vi "ERROR HANDLER.vi"(2 "error in":T1, 3 "GPIB address":string="8") -> (0 "error out":T1, 1 "error found":bool)   [LabVIEW 2025, in "MyDS360.lvlib"]
doc: "This support subVI queries the instrument's event status bit #4 which reports an execution error .\n ERROR FOUND is set to TRUE when an out of range parameter causes an execution error . \n This subVI is used in the function subVIs after setting some or all of the instrument's functions .\n The status of ERROR FOUND is then used in the function subVIs to report an error for the parameter that caused it ."
uses:
  MyDS360.lvlib
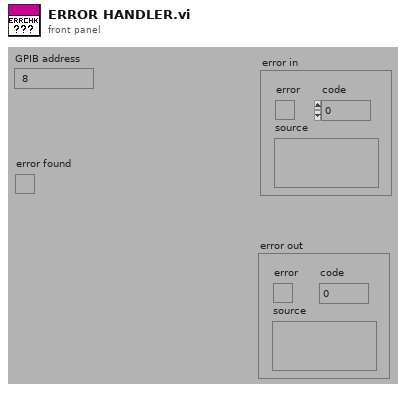
[diagram p1: front panel]
types:
  T1 = cluster{"error":bool, "code":i32, "source":string}
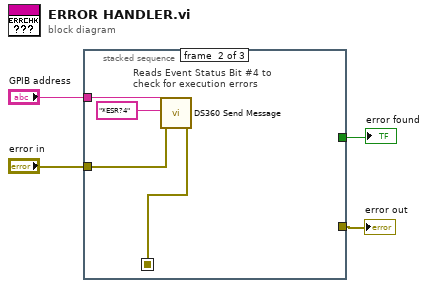
[diagram p0: block diagram]
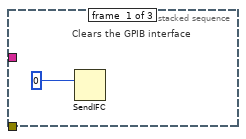
[diagram p2: hidden frame]
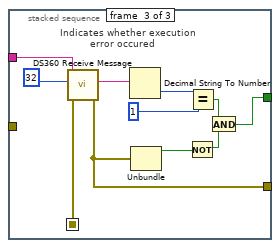
[diagram p3: hidden frame]
diagram:
  n1 = stacked-sequence {
    seq-local: [_ w8 _] -> [_ _ w20]
    tunnel: "GPIB address" -> [_ w9 w19]
    tunnel: "error in" -> [_ w7 _]
    tunnel: [_ _ w12] -> w2
    tunnel: [_ _ w10] -> w1
    frame #0 {
      # "Clears the GPIB interface"
      n2 = SendIFC(3:0) -> ()  [unwired: 1 in, 2 out]
    }
    frame #1 {
      # "Reads Event Status Bit #4 to                                                    check for execution errors"
      n3 = call "DS360 Send Message.vi"("address string"=w9, "write buffer"="*ESR?4", "error in"=w7) -> ("error out"=w8:T1)  [unwired: 3 in, 3 out]
    }
    frame #2 {
      # "Indicates whether execution \n          error occured"
      n4 = call "DS360 Receive Message.vi"("address string"=w19, "byte count"=32, "error in"=w20) -> ("read buffer"=w11:string, "error out"=w12:T1)  [unwired: 3 in, 2 out]
      n5 = Decimal String To Number(string=w11) -> (number=w17:i32)  [unwired: 2 in, 1 out]
      n6 = Unbundle(w12) -> ("error"=w15:bool)  [unwired: 2 out]
      n7 = Not(x=w15) -> (.not. x?=w14:bool)
      n8 = Equal?(x=w17, y=1) -> (x = y?=w13:bool)
      n9 = And(x=w13, y=w14) -> (x .and. y?=w10:bool)
    }
  }
  "error out" <- w2
  "error found" <- w1
